vi "Expand_Iterations.vi"(1 "Input Sequence":cluster{string, string[], dbl[], dbl}[](array[cluster])) -> (0 "Output Sequence":cluster{string, string[], dbl[], dbl}[](array[cluster]))   [LabVIEW 2011]
doc: "Expands all events in the sequence according to their \"Iterations\" argument, excluding loops. For example, an event with 3 iterations will be copied into 3 separate events."
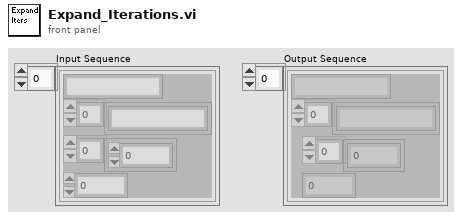
[diagram p1: front panel]
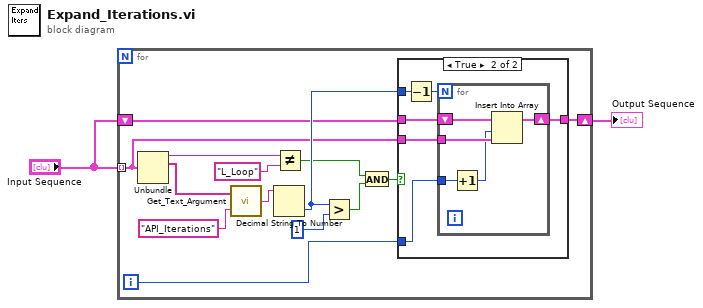
[diagram p0: block diagram]
diagram:
  n1 = for {
    tunnel: "Input Sequence" -> [w9] mode=indexing
    shift-right: [w8] -> w1
    shift-left: "Input Sequence" -> [w10]
    i -> [w11]
    n2 = Unbundle(w9) -> (w7:string, w12:string[])  [unwired: 2 out]
    n3 = call "Get_Text_Argument.vi"("Argument"="API_Iterations", "Argument List"=w12) -> ("Text"=w15:string)
    n4 = Decimal String To Number(string=w15) -> (number=w14:i32)  [unwired: 2 in, 1 out]
    n5 = Not Equal?(x=w7, y="L_Loop") -> (x != y?=w4:bool)
    n6 = Greater?(x=w14, y=1) -> (0:w5:bool)
    n7 = And(x=w4, y=w5) -> (x .and. y?=w3:bool)
    n8 = case shown="True" w3 {
      tunnel: w14 -> [_ w19]
      tunnel: w11 -> [_ w23]
      tunnel: [w17 w20] -> w8
      tunnel: w10 -> [w17 w22]
      tunnel: w9 -> [_ w21]
      frame False {
      }
      frame True {
        n9 = Decrement(x=w19) -> (x-1=w18:i32)
        n10 = for {
          N: w18 -> [_]
          shift-right: [w27] -> w20
          shift-left: w22 -> [w28]
          tunnel: w23 -> [w25]
          tunnel: w21 -> [w26]
          n11 = Increment(x=w25) -> (x+1=w24:i32)
          n12 = Insert Into Array(array=w28, index=w24, new element=w26) -> (w27:cluster{string, string[], dbl[], dbl}[])
        }
      }
    }
  }
  "Output Sequence" <- w1
